vi "comunication clusters.vi"() -> (3 "DS to robot 2":T3)   [LabVIEW 2016]
uses:
  Auto modes.ctl
  Shifter override.ctl
panel:
  in  "DS to robot":T3
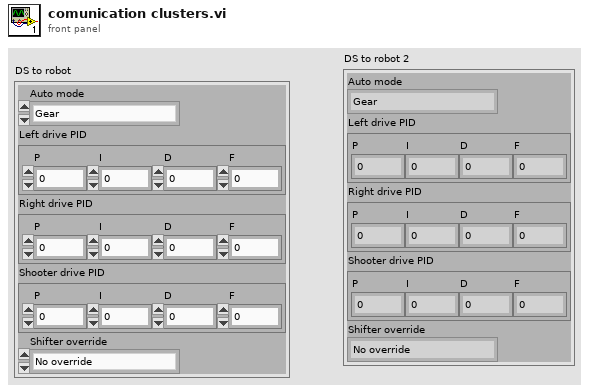
[diagram p1: front panel]
types:
  T1 = typedef "Auto modes.ctl" = enum16{"Gear", "Shooter", "Gear + Shooter", "None", "Shooter + Cheesecake", "Shooter + Bin"}
  T2 = typedef "Shifter override.ctl" = enum16{"No override", "High ", "Low"}
  T3 = cluster{"Auto mode":T1, "Left drive PID ":cluster{"P":dbl, "I":dbl, "D":dbl, "F":dbl}, "Right drive PID ":cluster{"P":dbl, "I":dbl, "D":dbl, "F":dbl}, "Shooter drive PID ":cluster{"P":dbl, "I":dbl, "D":dbl, "F":dbl}, "Shifter override":T2}
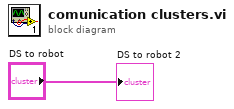
[diagram p0: block diagram]
diagram:
  "DS to robot 2" <- "DS to robot"
